vi "Get Glyph Index.vi"(9 "URL":string, 10 "Type":string, 11 "LV Proj File Path":path) -> (2 "Glyph Index":i32)   [LabVIEW 2016]
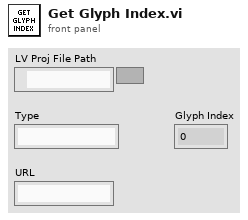
[diagram p1: front panel]
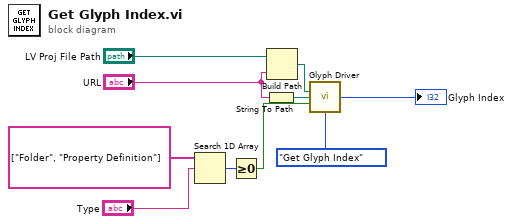
[diagram p0: block diagram]
diagram:
  n1 = Search 1D Array(1D array=string[] ["Folder", "Property Definition"], element="Type") -> (index of element=w2:i32)  [unwired: 1 in]
  n2 = Greater Or Equal To 0?(x=w2) -> (x >= 0?=w1:bool)
  n3 = String To Path(string="URL") -> (path=w8:path)
  n4 = Build Path(base path="LV Proj File Path", name or relative path="URL") -> (appended path=w10:path)
  n5 = call "Glyph Driver.vi"("File Path"=w10, "File Relative Path"=w8, "Is Folder?"=w1, "Op Mode"=enum16{"Get Glyph Index", "Get all Glyphs"}."Get Glyph Index") -> ("Glyph Index"=→"Glyph Index":i32)  [unwired: 9 in, 2 out]
